vi "Pi_Main - STM.vi"   [LabVIEW 2014]
uses:
  <vilib>/NI/STM/SubVIs/MetaDataElement.ctl
  <vilib>/NI/STM/TCP/TCP Write Options.ctl
  <vilib>/Analysis/4window.llb/windowTd.ctl
  <vilib>/MakerHub/LINX/Public/Peripherals/Digital/Digital Write 1 Chan.vi
  <vilib>/NI/STM/TCP/Write Meta Data (TCP Ref).vi
  <vilib>/NI/STM/TCP/Get Connection Reference (TCP).vi
  <vilib>/MakerHub/LINX/Public/Peripherals/Digital/Digital Write N Chans.vi
  <vilib>/MakerHub/LINX/Private/Local IO/LinxDigitalWrite.vi
  <vilib>/MakerHub/LINX/Public/Utilities/Check Channel.vi
  <vilib>/MakerHub/LINX/Private/Local IO/Handle Errors.vi
  <vilib>/Utility/error.llb/Error Cluster From Error Code.vi
  <vilib>/MakerHub/LINX/Public/Utilities/Open Local.vi
  <vilib>/MakerHub/LINX/Private/Utilties/Generate Error.vi
  <vilib>/NI/STM/TCP/Write Meta Data (TCP Clst).vi
  <vilib>/NI/STM/TCP/Write Message (TCP).vi
  <vilib>/measure/maspectr.llb/FFT Power Spectrum and PSD for 1 Chan (CDB).vi
  <vilib>/ErrorRing/Error Ring.xnode
  <vilib>/measure/NI_MAPro.lvlib
  <vilib>/Analysis/NI_AALPro.lvlib
  <vilib>/NI/STM/NI STM.lvlib
  <vilib>/MakerHub/LINX/LMH-LINX.lvlib
types:
  T1 = typedef "NI STM.lvlib/TCP Write Options.ctl" = cluster{"ignore timeout error":bool, "timeout ms (1000)":i32}
  T2 = typedef "NI STM.lvlib/MetaDataElement.ctl" = string
  T3 = typedef "NI STM.lvlib/TCP Connection Info.ctl" = cluster{"connection ID":refnum<k5>, "meta data":T2[]}
  T4 = typedef "LMH-LINX.lvlib/LINX Ref.ctl" = cluster{"IO":T5, "Interface":T6, "LINX Device Config":T7}
  T5 = typedef "LMH-LINX.lvlib/Platform.ctl" = enum16{"Remote", "Local"}
  T6 = typedef "LMH-LINX.lvlib/Interface.ctl" = enum16{"Serial", "TCP"}
  T7 = typedef "LMH-LINX.lvlib/Device.lvlib/LINX Device Config.ctl" = cluster{"Interface":T6, "COM Port":refnum<visa-resource-name>, "TCP Configuration":T8, "Device Family":u8, "Device ID":u8, "Device Name":string, "TCP Ref":refnum<k5>, "Channels":T9}
  T8 = typedef "LMH-LINX.lvlib/Device.lvlib/TCP Config.ctl" = cluster{"IP Address":string, "Port":u16}
  T9 = typedef "LMH-LINX.lvlib/Channels.ctl" = cluster{"DI":u8[], "DO":u8[], "AI":u8[], "AO":u8[], "PWM":u8[], "QE":u8[], "UART":u8[], "I2C 2":u8[], "SPI":u8[], "CAN":u8[], "Servo":u8[], "AI Ref (V)":dbl, "AI Resolution (Bits)":u8, "AO Ref (V)":dbl, "AO Resolution (Bits)":u8}
  T10 = typedef "NI_AALPro.lvlib/windowTd.ctl" = u32
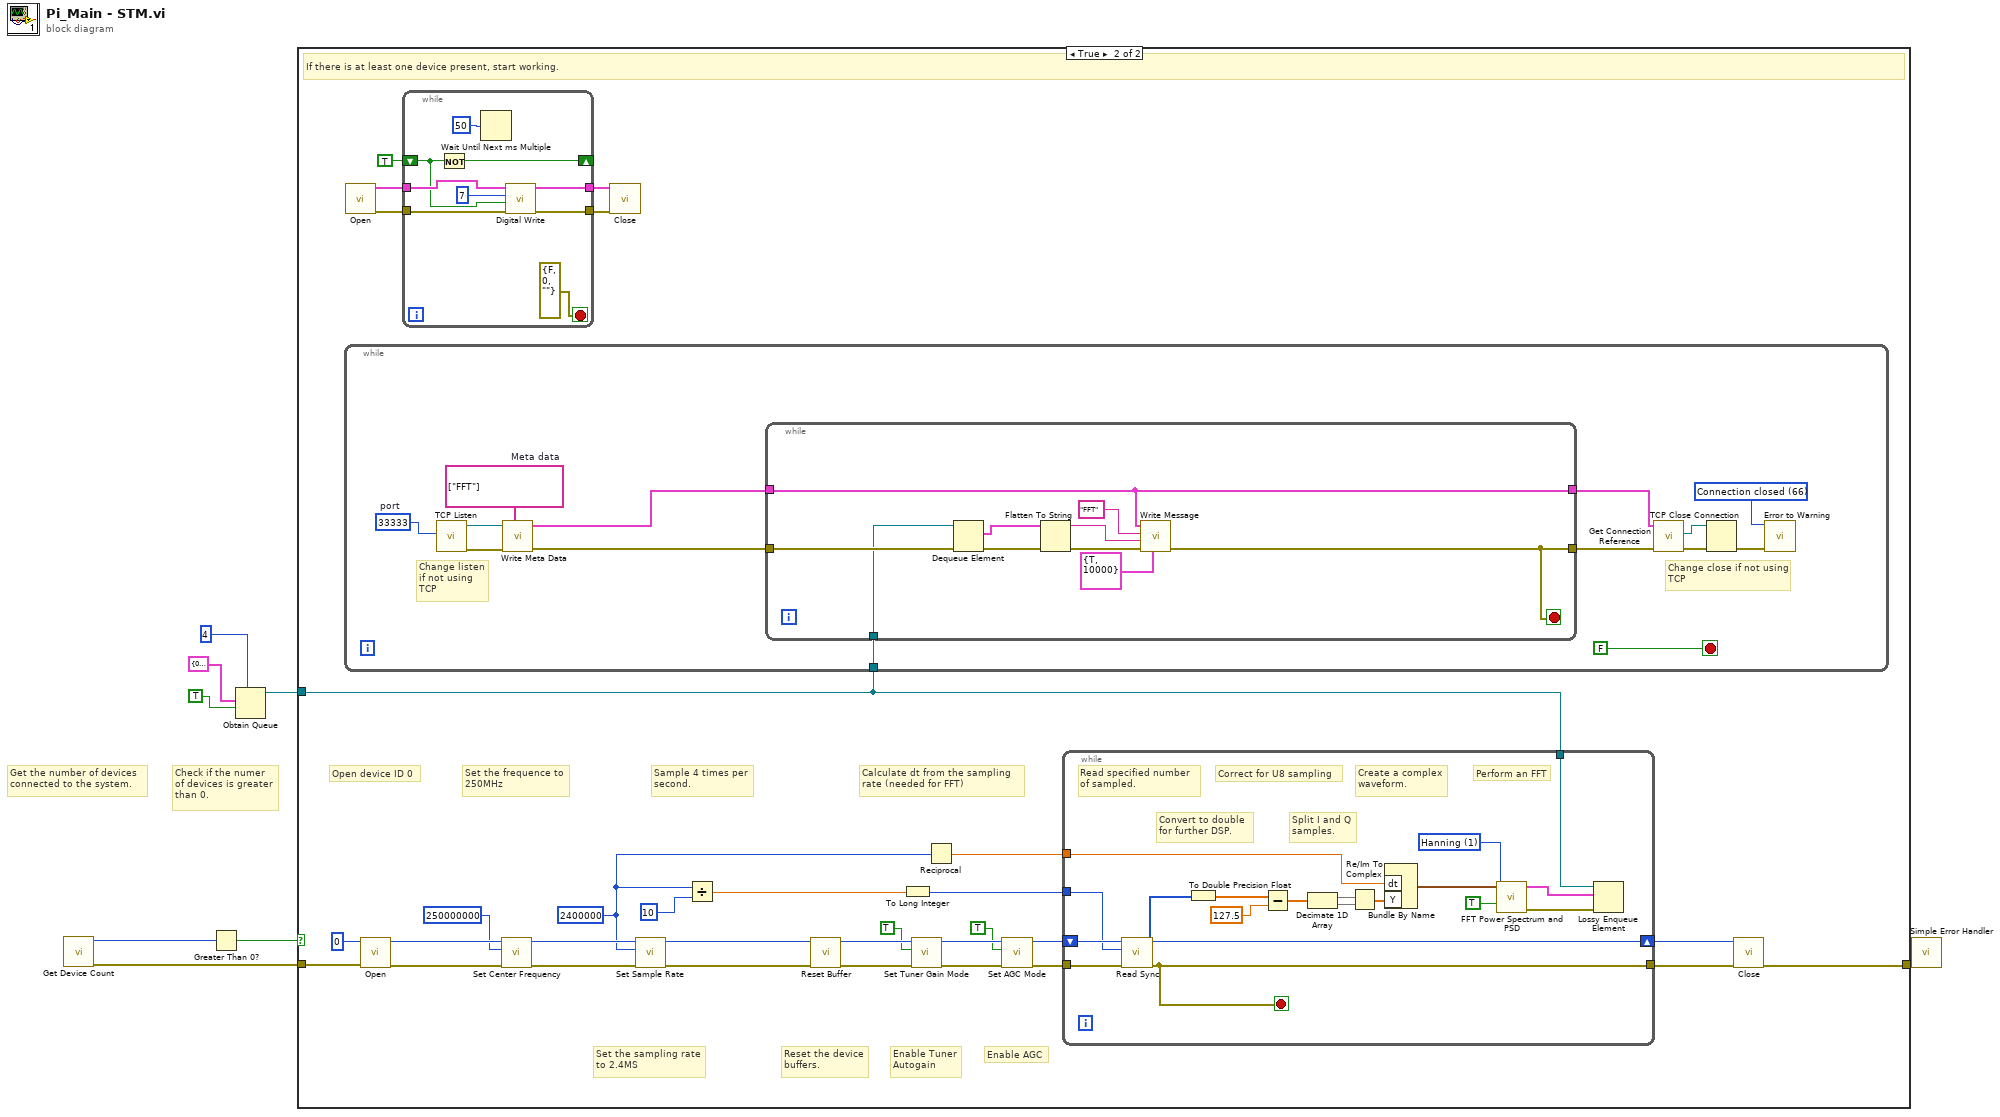
[diagram p0: block diagram]
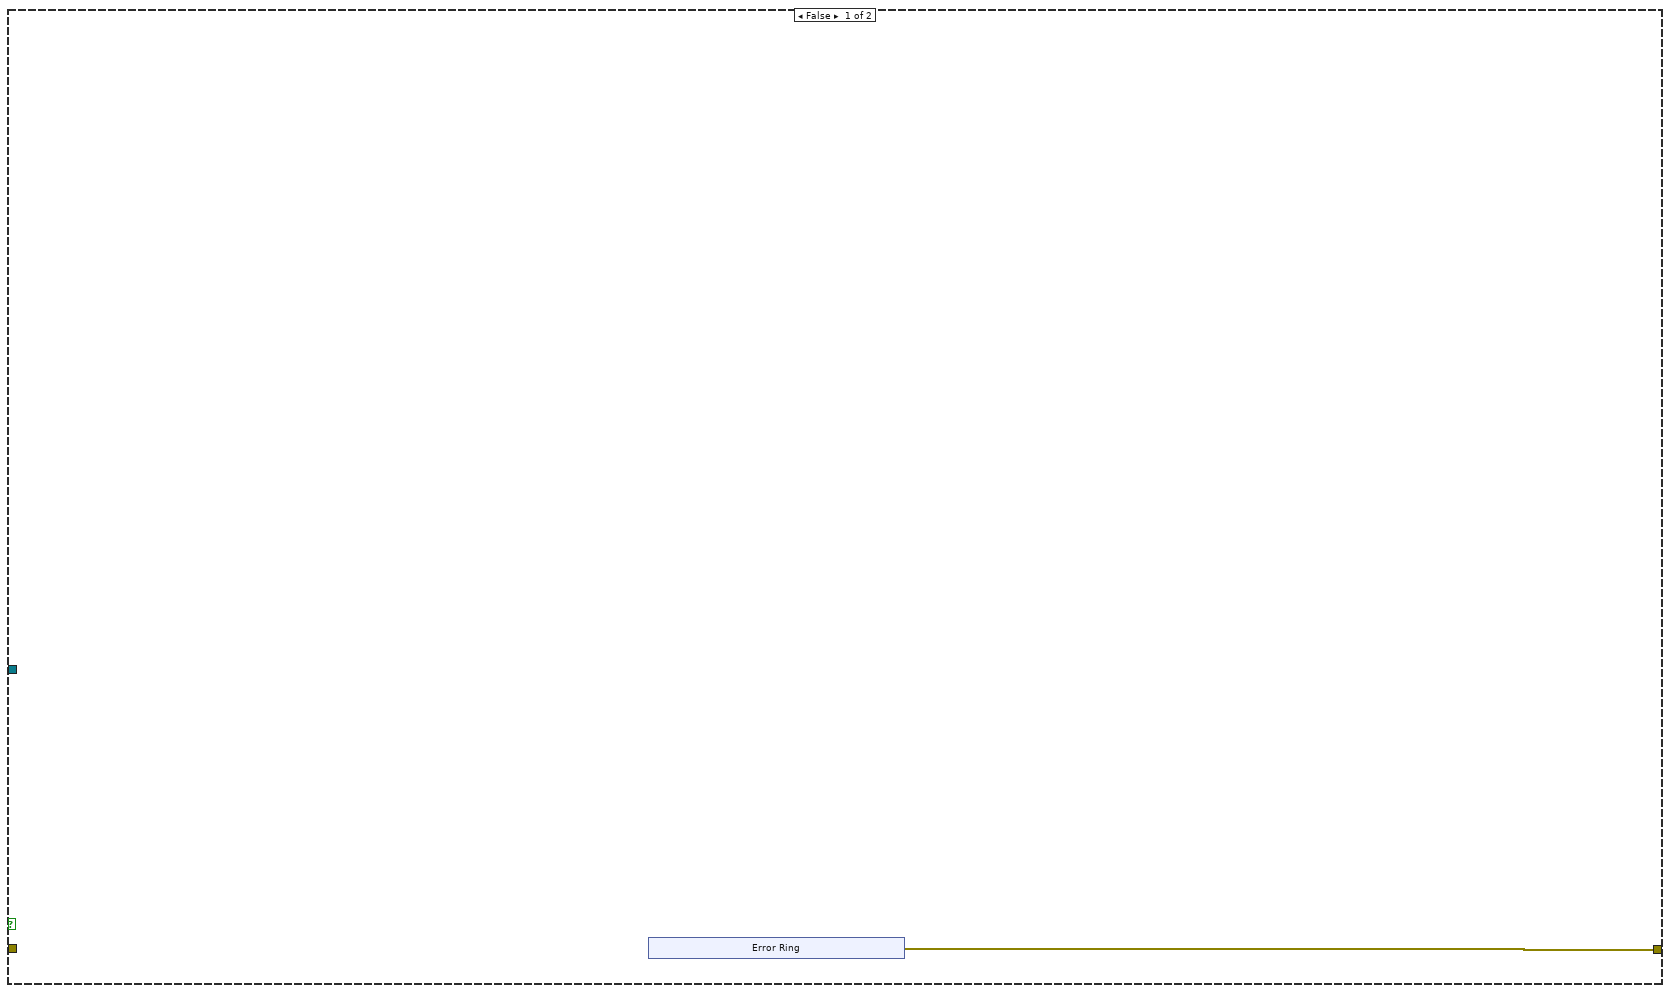
[diagram p2: hidden frame]
diagram:
  # "Check if the numer\nof devices is greater\nthan 0."
  # "Get the number of devices\nconnected to the system."
  n1 = call "Get Device Count.vi"() -> ("error out"=w5:errorcluster, "Device Count"=w8:u32)  [unwired: 10 in]
  n2 = Greater Than 0?(x=w8) -> (x > 0?=w7:bool)
  n3 = Obtain Queue(max queue size (-1, unlimited)=4, element data type=cluster{"f0":dbl, "df":dbl, "magnitude":dbl[]} {"f0"=0.0, "df"=0.0, "magnitude"=[]} ("Power Spectrum / PSD"), create if not found? (T)=TRUE) -> (queue out=w1:refnum<queue>)  [unwired: 2 in, 2 out]
  n4 = case shown="True" w7 {
    tunnel: w5 -> [_ w44]
    tunnel: [w9 w27] -> w6
    tunnel: w1 -> [_ w19]
    frame False {
      n5 = xnode "Error Ring"() -> ("error out"=w9:errorcluster)
    }
    frame True {
      w22 = u32 2400000 ("Sample Rate")
      # "Sample 4 times per\nsecond."
      # "Calculate dt from the sampling\nrate (needed for FFT)"
      # "Enable AGC"
      # "Enable Tuner\nAutogain"
      # "Reset the device\nbuffers."
      # "Set the sampling rate\nto 2.4MS"
      # "Set the frequence to\n250MHz"
      # "Open device ID 0"
      # "If there is at least one device present, start working."
      n6 = while {
        tunnel: w19 -> [w67]
        stop <- FALSE stop-if-true
        w60 = 66 items=["No Error", "Argument Error", "Memory Full", "Out of Zone", "End of File", "File Already Open", "Generic File IO Error", "File Not Found", "File Permission Error", "Disk Full", "Duplicate Path", "Too Many Files Open", "Not Enabled", "Resource File Not Found", "Cannot Add Resource", "Resource Not Found", "Image Not Found", "Image Memory Error", "Pen Does Not Exist", "Config Bad Type", "Config Token Not Found", "Config Parse Error", "Config Memory Error", "Bad External Code Format", "Bad External Code Offset", "External Code Not Present", "Null Window", "Destroy Window Mixup", "Null Menu", "Print Aborted", "Bad Print Record", "Print Driver Error", "Windows Error During Print", "Memory Error During Print", "Print Dialog Error", "Generic Print Error", "Invalid Device Refnum", "Device Not Found", "Device Parameter Error", "Device Unit Error", "Can't Open Device", "Device Call Aborted", "Generic Error", "Cancelled By User", "Object ID Too Low", "Object ID Too High", "Object Not In Heap", "Unknown Heap", "Bad DefProc ID", "DefProc Not In Table", "Message Out Of Range", "Null Method", "Unknown Message", "Manager Call Not Supported", "Bad address", "Connection In progress", "Connection timed out", "Connection is already in progress", "Network attribute not supported", "Network error", "Address in use", "System out of memory", "Connection aborted", "Connection refused", "Connection is not connected", "Connection is already connected", "Connection closed", "Initialize error (interapplication manager)", "Bad occurrence", "Wait on unbound occurrence handler", "Occurrence queue overflow", "Bad path", "Semaphore not signaled", "Unrecognized type (interapplication manager)"] ("1st Error to Convert")
        w64 = T2[] ["FFT"]  # Meta data
        w62 = u16 33333  # port
        # "Change close if not using TCP"
        # "Change listen if not using TCP"
        n7 = call <vilib>:"TCP Listen.vi"("port"=w62) -> ("error out"=w63:errorcluster, "connection ID"=w65:refnum<k5>)  [unwired: 3 in, 6 out]
        n8 = call-poly <vilib>:"Write Meta Data.vi"("meta data"=w64, "error in"=w63, "connection ID"=w65) -> ("error out"=w54:errorcluster, "connection info out"=w55:T3)  [unwired: 2 in, 5 out]
        n9 = while {
          tunnel: w54 -> [w70]
          tunnel: w67 -> [w68]
          tunnel: w55 -> [w76]
          tunnel: [w77] -> w56
          tunnel: [w76] -> w57
          stop <- w77 stop-if-true
          n10 = Dequeue Element(queue=w68, error in (no error)=w70) -> (element=w69:cluster{"f0":dbl, "df":dbl, "magnitude":dbl[]}, error out=w71:errorcluster)  [unwired: 1 in, 2 out]
          n11 = Flatten To String(anything=w69, error in (no error)=w71) -> (data string=w74:string, error out=w75:errorcluster)  [unwired: 2 in, 1 out]
          n12 = call-poly <vilib>:"Write Message.vi"("options"=T1 {"ignore timeout error"=TRUE, "timeout ms (1000)"=10000}, "error in"=w75, "data"=w74, "name"="FFT", "connection info in"=w76) -> ("error out"=w77:errorcluster)  [unwired: 5 in, 1 out]
        }
        n13 = call-poly <vilib>:"Get Connection Reference.vi"("error in"=w56, "connection info in"=w57) -> ("error out"=w59:errorcluster, "connection ID out"=w58:refnum<k5>)  [unwired: 8 out]
        n14 = TCP Close Connection(connection ID=w58, error in (no error)=w59) -> (error out=w61:errorcluster)  [unwired: 2 out]
        n15 = call <vilib>:"Error to Warning.vi"("1st Error to Convert"=w60, "error in"=w61) -> ()  [unwired: 3 in, 11 out]
      }
      n16 = call-poly <vilib>:"Open.vi"() -> ("Error Out"=w17:errorcluster, "LINX Resource"=w18:T4)  [unwired: 9 in, 1 out]
      n17 = call <vilib>:"Open.vi"("error in (no error)"=w44, "Device Index"=u32 0) -> ("error out"=w41:errorcluster, "DeviceRefnum Out"=w42:u64)  [unwired: 6 in]
      n18 = while {
        tunnel: w18 -> [w53]
        tunnel: w17 -> [w52]
        tunnel: [w46] -> w16
        tunnel: [w51] -> w15
        shift-right: [w49] -> _
        shift-left: TRUE -> [w48]
        stop <- errorcluster {"status"=FALSE, "code"=0, "source"=""} ("error IO") stop-if-true
        n19 = Not(x=w48) -> (.not. x?=w49:bool)
        n20 = Wait Until Next ms Multiple(millisecond multiple=u32 50) -> ()  [unwired: 1 out]
        n21 = call-poly <vilib>:"Digital Write.vi"("Error In"=w52, "Output Value"=w48, "DO Channel"=u8 7, "LINX Resource"=w53) -> ("Error Out"=w46:errorcluster, "LINX Resource"=w51:T4)  [unwired: 6 in]
      }
      n22 = call "Set Center Frequency.vi"("error in (no error)"=w41, "Center Frequency"=u32 250000000, "DeviceRefnum"=w42) -> ("error out"=w40:errorcluster, "DeviceRefnum Out"=w39:u64)  [unwired: 6 in, 1 out]
      n23 = call <vilib>:"Close.vi"("Error In"=w16, "LINX Resource"=w15) -> ()  [unwired: 9 in, 1 out]
      n24 = call "Set Sample Rate.vi"("error in (no error)"=w40, "Sample Rate"=w22, "DeviceRefnum"=w39) -> ("error out"=w20:errorcluster, "DeviceRefnum Out"=w38:u64)  [unwired: 6 in, 1 out]
      n25 = Divide(x=w22, y=u32 10) -> (x/y=w23:dbl)
      n26 = call "Reset Buffer.vi"("error in (no error)"=w20, "DeviceRefnum"=w38) -> ("error out"=w36:errorcluster, "DeviceRefnum Out"=w37:u64)  [unwired: 7 in, 1 out]
      n27 = To Long Integer(number=w23) -> (32bit integer=w24:i32)
      n28 = call "Set Tuner Gain Mode.vi"("error in (no error)"=w36, "AutoGain"=TRUE, "DeviceRefnum"=w37) -> ("error out"=w34:errorcluster, "DeviceRefnum Out"=w33:u64)  [unwired: 6 in, 1 out]
      n29 = Reciprocal(x=w22) -> (1/x=w26:dbl)
      n30 = call "Set AGC Mode.vi"("error in (no error)"=w34, "AGC Enable"=TRUE, "DeviceRefnum"=w33) -> ("error out"=w31:errorcluster, "DeviceRefnum Out"=w30:u64)  [unwired: 6 in, 1 out]
      n31 = while {
        tunnel: w31 -> [w96]
        shift-right: [w94] -> w29
        shift-left: w30 -> [w95]
        tunnel: [w78] -> w28
        tunnel: w26 -> [w88]
        tunnel: w24 -> [w84]
        tunnel: w19 -> [w81]
        stop <- w78 stop-if-true
        w86 = T10 1 items=["Rectangle"=0, "Hanning"=1, "Hamming"=2, "Blackman-Harris"=3, "Exact Blackman"=4, "Blackman"=5, "Flat Top"=6, "4 Term B-Harris "=7, "7 Term B-Harris"=8, "Low Sidelobe"=9, "Blackman Nuttall"=11, "Triangle"=30, "Bartlett-Hanning"=31, "Bohman"=32, "Parzen"=33, "Welch"=34, "Kaiser"=60, "Dolph-Chebyshev"=61, "Gaussian"=62] ("window")
        # "Perform an FFT"
        # "Convert to double\nfor further DSP."
        # "Split I and Q\nsamples."
        # "Correct for U8 sampling"
        # "Create a complex\nwaveform."
        # "Read specified number\nof sampled."
        n32 = call "Read Sync.vi"("error in (no error)"=w96, "Number Of Samples"=w84, "DeviceRefnum"=w95) -> ("error out"=w78:errorcluster, "Sample Buffer"=w83:u8[], "DeviceRefnum Out"=w94:u64)  [unwired: 5 in, 1 out]
        n33 = To Double Precision Float(number=w83) -> (double precision float=w93:dbl[])
        n34 = Subtract(x=w93, y=127.5) -> (x-y=w92:dbl[])
        n35 = Decimate 1D Array(w92) -> (w91:dbl[], w90:dbl[])
        n36 = Re/Im To Complex(1:w90, 2:w91) -> (0:w82:cdb[])
        n37 = Bundle By Name("dt"=w88, "Y"=w82) -> (w87:waveform(cdb))  [unwired: 1 in]
        n38 = call-poly <vilib>:"FFT Power Spectrum and PSD.vi"("dB On (F)"=TRUE, "window"=w86, "time signal"=w87) -> ("error out"=w80:errorcluster, "Power Spectrum / PSD"=w79:cluster{"f0":dbl, "df":dbl, "magnitude":dbl[]})  [unwired: 5 in, 2 out]
        n39 = Lossy Enqueue Element(queue=w81, element=w79, error in (no error)=w80) -> ()  [unwired: 4 out]
      }
      n40 = call <vilib>:"Close.vi"("error in (no error)"=w28, "DeviceRefnum"=w29) -> ("error out"=w27:errorcluster)  [unwired: 8 in, 1 out]
    }
  }
  n41 = call <vilib>:"Simple Error Handler.vi"("error in (no error)"=w6) -> ()  [unwired: 4 in, 5 out]
